vi "Set_Rescaling_Setting.vi"(6 "isOriginalMonitor":bool, 8 "error in (no error)":errorcluster, 9 "avg":dbl, 10 "mode":i32(ring) items=["Freerun_SPU", "Freerun_Referencemodule"], 11 ".NET Reference in":refnum<k24>) -> (0 "error out":errorcluster, 3 "Reference out":refnum<k24>)   [LabVIEW 2017]
doc: "Setting for STS rescaling mode"
uses:
  D:/test/PDLSTS/LV_PDL LvVer17.0/LV_PDL_x64/DLL/STSProcess.dll
  DLL/STSProcess.dll
  Share/MPM_PowerMonitorType.vi
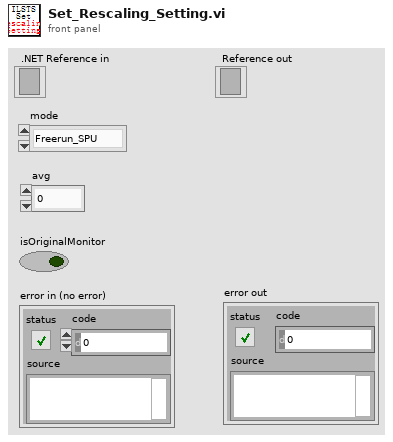
[diagram p1: front panel]
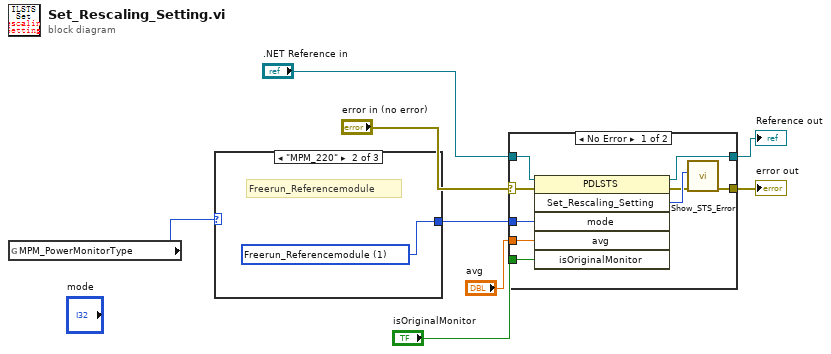
[diagram p0: block diagram]
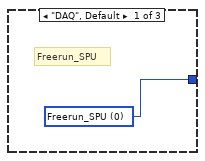
[diagram p2: hidden frame]
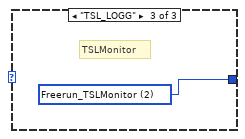
[diagram p3: hidden frame]
diagram:
  n1 = global read "MPM_PowerMonitorType.vi" "MPM_PowerMonitorType"() -> (w1:enum16{"DAQ", "MPM_220", "TSL_LOGG"})
  n2 = case shown="\"MPM_220\"" w1 {
    tunnel: [w9 w10 w11] -> w2
    frame "DAQ", Default {
      w9 = 0 items=["Freerun_SPU", "Freerun_Referencemodule", "Freerun_TSLMonitor"] ("mode")
      # "Freerun_SPU"
    }
    frame "MPM_220" {
      w10 = 1 items=["Freerun_SPU", "Freerun_Referencemodule", "Freerun_TSLMonitor"] ("mode")
      # "Freerun_Referencemodule"
    }
    frame "TSL_LOGG" {
      w11 = 2 items=["Freerun_SPU", "Freerun_Referencemodule", "Freerun_TSLMonitor"] ("mode")
      # "TSLMonitor"
    }
  }
  n3 = case shown="No Error" "error in (no error)" {
    selector: "error in (no error)" -> [w18 w22]
    tunnel: ".NET Reference in" -> [w20 w21]
    tunnel: [w19 w21] -> w8
    tunnel: [w15 w22] -> w6
    tunnel: w2 -> [w14 _]
    tunnel: "avg" -> [w13 _]
    tunnel: "isOriginalMonitor" -> [w12 _]
    frame No Error {
      n4 = invoke on="调用节点" class="PDLSTS" method="Set_Rescaling_Setting"(reference=w20, error in=w18, "mode"=w14, "avg"=w13, "isOriginalMonitor"=w12) -> (reference out=w19:refnum<k24>, error out=w16:errorcluster, "Set_Rescaling_Setting"=w17:i32)  [unwired: 1 in, 3 out]
      n5 = call "Show_STS_Error.vi"("error in (no error)"=w16, "Error"=w17) -> ("error out"=w15:errorcluster)  [unwired: 9 in]
    }
    frame Error {
    }
  }
  "error out" <- w6
  "Reference out" <- w8
